vi "Read Measurement Simultaneously.vi"(8 "Error In (no error)":errorcluster, 10 "Parameters (0: X, 1: Y)":i32[](array[ring])=[0, 1] items=["X", "Y", "R [V]", "R [dBm]", "Phi", "AUX IN 1", "AUX IN 2", "Reference Frequency", "CH1 Display", "CH2 Display"], 11 "VISA Resource Name":refnum<visa-resource-name>) -> (0 "Error Out":errorcluster, 2 "Values":dbl[](array[numeric]) format="%.2e", 3 "VISA Resource Name Out":refnum<visa-resource-name>)   [LabVIEW 2010, in "Stanford Research 844.lvlib"]
doc: "This VI reads the values of up to six parameters at a single instant.\n\nNote: The values of X and Y are recorded at a single instant, as are the values of R[V] and Phi. Thus reading (X,Y) or (R,Phi) yields a snapshot of the input signal. A measurement of X, Y, R and Phi may give R,Phi measured at a time up to 84 µs before\nthe X,Y measurement.\nR[dBm] and the Aux Inputs are computed with a maximum interval of 84 µs. A measurement of X, Y, and AUX IN 1 will give AUX IN 1 measured at a time up to 84 µs before the X,Y measurement.\nThe reference frequency is computed 6-12 times a second."
uses:
  <instrlib>/Stanford Research 844/Stanford Research 844.lvlib
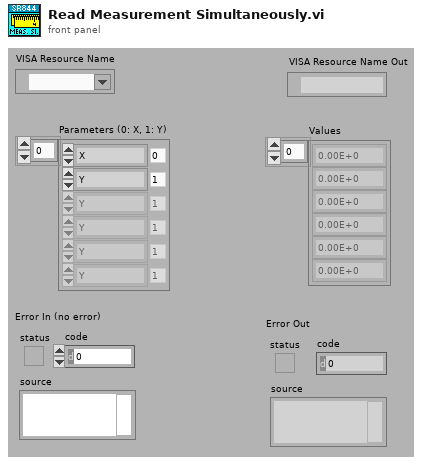
[diagram p1: front panel]
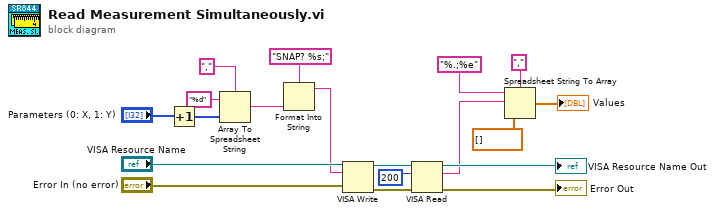
[diagram p0: block diagram]
diagram:
  n1 = Increment(x="Parameters (0: X, 1: Y)") -> (x+1=w2:i32[])
  n2 = Array To Spreadsheet String(delimiter (Tab)=",", array=w2, 3:"%d" ("format string")) -> (spreadsheet string=w4:string)
  n3 = Format Into String(format string="SNAP? %s;", w4) -> (resulting string=w1:string)  [unwired: 2 in, 1 out]
  n4 = VISA Write(VISA resource name="VISA Resource Name", write buffer=w1, error in (no error)="Error In (no error)") -> (VISA resource name out=w17:refnum<visa-resource-name>, error out=w16:errorcluster)  [unwired: 1 out]
  n5 = VISA Read(VISA resource name=w17, byte count=u32 200 ("byte count (0)"), error in (no error)=w16) -> (VISA resource name out=→"VISA Resource Name Out":refnum<visa-resource-name>, read buffer=w12:string, error out=→"Error Out":errorcluster)  [unwired: 1 out]
  n6 = Spreadsheet String To Array(delimiter (Tab)=",", format string="%.;%e", spreadsheet string=w12, array type (2D Dbl)=dbl[] []) -> (array=→"Values":dbl[])
